vi "Global Sensors.vi"() -> ()   [LabVIEW 2019, in "Untitled Library 1.lvlib"]
uses:
  Untitled Library 1.lvlib
panel:
  in  "Top":bool
  in  "Invert Intake":bool
  in  "State":enum16{"Lemon", "Roulette", "Climb"}(ring)=enum."Climb"
  in  "Match Time":dbl
  in  "Lemon State":enum16{"Intake", "Clear shooter", "Shoot"}(ring)=enum."Clear shooter"
  in  "FMS":string
  in  "ColorSensor":string
  in  "Bot":bool
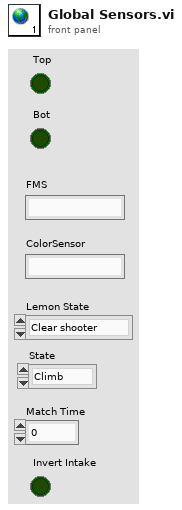
[diagram p1: front panel]
diagram:
